vi "reBuildJoindCommand.vi"(2 "number of group elements (0)":i32, 3 "Args":string[](array[string]), 4 "Command 2":string) -> (0 "Arg":string, 1 "Command":string)   [LabVIEW 2011]
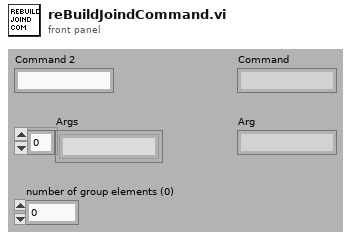
[diagram p1: front panel]
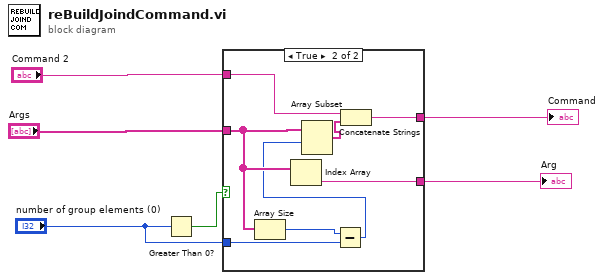
[diagram p0: block diagram]
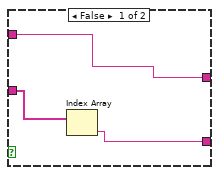
[diagram p2: hidden frame]
diagram:
  n1 = Greater Than 0?(x="number of group elements (0)") -> (x > 0?=w5:bool)
  n2 = case shown="True" w5 {
    tunnel: "Command 2" -> [w9 w17]
    tunnel: "Args" -> [w8 w13]
    tunnel: [w9 w16] -> w3
    tunnel: [w7 w15] -> w4
    tunnel: "number of group elements (0)" -> [_ w14]
    frame False {
      n3 = Index Array(array=w8) -> (element=w7:string)  [unwired: 1 in]
    }
    frame True {
      n4 = Array Size(array=w13) -> (size(s)=w12:i32)
      n5 = Index Array(array=w13) -> (element=w15:string)  [unwired: 1 in]
      n6 = Subtract(x=w12, y=w14) -> (x-y=w11:i32)
      n7 = Array Subset(array=w13, index=w11) -> (w10:string[])  [unwired: 1 in]
      n8 = Concatenate Strings(w17, w10) -> (w16:string)
    }
  }
  "Arg" <- w4
  "Command" <- w3
